vi "DMA.Command.Handler.vi"(10 "DMA.Enable":bool, 11 "DMA.MinimumSamples":u32) -> (3 "Transfer":bool)   [LabVIEW 2015]
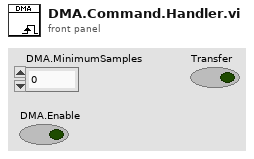
[diagram p1: front panel]
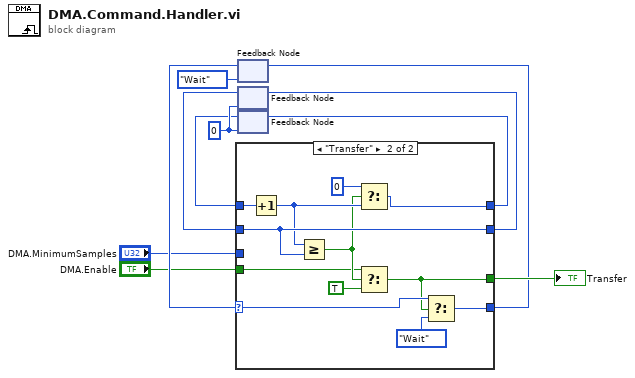
[diagram p0: block diagram]
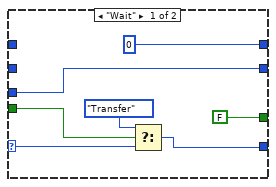
[diagram p2: hidden frame]
diagram:
  w6 = u32 0 ("t")
  n1 = feedback #1(enum8{"Wait", "Transfer"}."Wait") -> (w10:enum8{"Wait", "Transfer"})
  n2 = feedback #2(w6) -> (w7:u32)
  n3 = feedback #3(w6) -> (w4:u32)
  n4 = case shown="\"Transfer\"" w10 {
    selector: w10 -> [w17 w22]
    tunnel: "DMA.Enable" -> [w18 w23]
    tunnel: [w15 w20] -> w9
    tunnel: "DMA.MinimumSamples" -> [w14 _]
    tunnel: [w14 w29] -> w5
    tunnel: [u32 0 w27] -> w3
    tunnel: w4 -> [_ w30]
    tunnel: w7 -> [_ w29]
    tunnel: [FALSE ("f") w19] -> w11
    frame "Wait" {
      n5 = Select(t=enum8{"Wait", "Transfer"}."Transfer", s=w18, f=w17) -> (s? t:f=w15:enum8{"Wait", "Transfer"})
    }
    frame "Transfer" {
      n6 = Increment(x=w30) -> (x+1=w28:u32)
      n7 = Greater Or Equal?(x=w28, y=w29) -> (x >= y?=w25:bool)
      n8 = Select(t=u32 0, s=w25, f=w28) -> (s? t:f=w27:u32)
      n9 = Select(t=w23, s=w25, f=TRUE) -> (s? t:f=w19:bool)
      n10 = Select(t=w22, s=w19, f=enum8{"Wait", "Transfer"}."Wait" ("t")) -> (s? t:f=w20:enum8{"Wait", "Transfer"})
    }
  }
  "Transfer" <- w11
  n11 = feedback-in #1(w9) -> ()
  n12 = feedback-in #2(w5) -> ()
  n13 = feedback-in #3(w3) -> ()
